vi "2700 or not.vi"() -> (0 "AVE  (V)":dbl format="%#_8g")   [LabVIEW 2010]
uses:
  Instance           2 19Saved   2700 or not .vi
panel:
  out "Waveform Chart":ext(graph)
  in  "# points":dbl=1.0
  out "read buffer":string
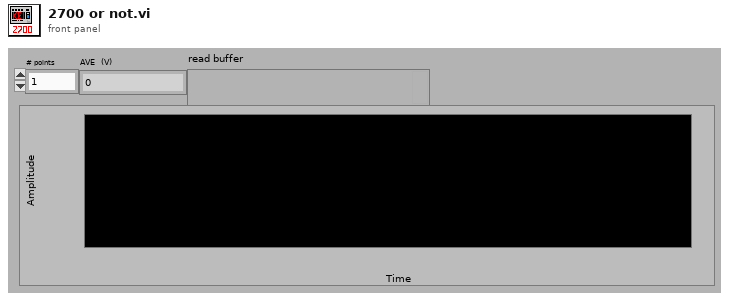
[diagram p1: front panel]
types:
  T1 = cluster{"error":bool, "code":i32, "source":string}
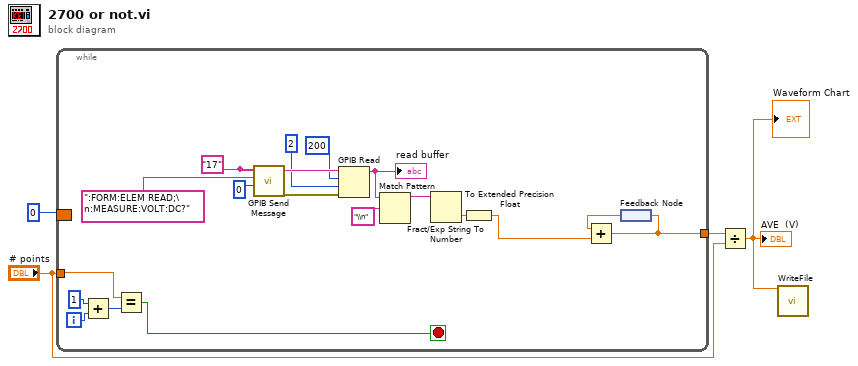
[diagram p0: block diagram]
diagram:
  n1 = while {
    tunnel: "# points" -> [w14]
    tunnel: [w6] -> w3
    border: 0 -> [_]
    i -> [w15]
    stop <- w13 stop-if-true
    w22 = "17" ("address string")
    n2 = Add(x=1, y=w15) -> (x+y=w5:i32)
    n3 = Equal?(x=w14, y=w5) -> (x = y?=w13:bool)
    n4 = call <instrlib>:"GPIB Send Message.vi"("address string"=w22, "write buffer"=":FORM:ELEM READ;\n:MEASURE:VOLT:DC?", "write mode (set END:0)"=0) -> ("error out"=w21:T1)  [unwired: 4 in, 2 out]
    n5 = GPIB Read(0:w22, 1:200 ("byte count"), 2:2, 3:w21) -> (5:w10:string)  [unwired: 1 in, 2 out]
    "read buffer" <- w10
    n6 = Match Pattern(string=w10, regular expression="\\n") -> (before substring=w11:string)  [unwired: 1 in, 3 out]
    n7 = Fract/Exp String To Number(string=w11) -> (number=w9:dbl)  [unwired: 3 in, 1 out]
    n8 = To Extended Precision Float(1:w9) -> (0:w8:ext)
    n9 = feedback #1() -> (w7:ext)
    n10 = Add(x=w7, y=w8) -> (x+y=w6:ext)
    n11 = feedback-in #1(w6) -> ()
  }
  n12 = Divide(x=w3, y="# points") -> (x/y=w1:ext)
  "AVE  (V)" <- w1
  "Waveform Chart" <- w1
  n13 = call "WriteFile"("Signals"=w1) -> ()  [unwired: 16 in, 3 out]
